vi "Serialize.vi"(0 "Input 6":variant, 4 "Input 5":variant, 6 "Input 4":variant, 8 "Input 3":variant, 9 "Input 2":variant, 10 "Input 1":variant, 11 "Base Actor in":refnum<class "Base Actor.lvclass">) -> (3 "Base Actor out":refnum<class "Base Actor.lvclass">)   [LabVIEW 2021, in "jettl.lvlib" / "Actor.lvlib" / "Base Actor.lvclass"]
uses:
  Base Actor.lvclass
  Base Actor.lvclass/Base Actor.ctl
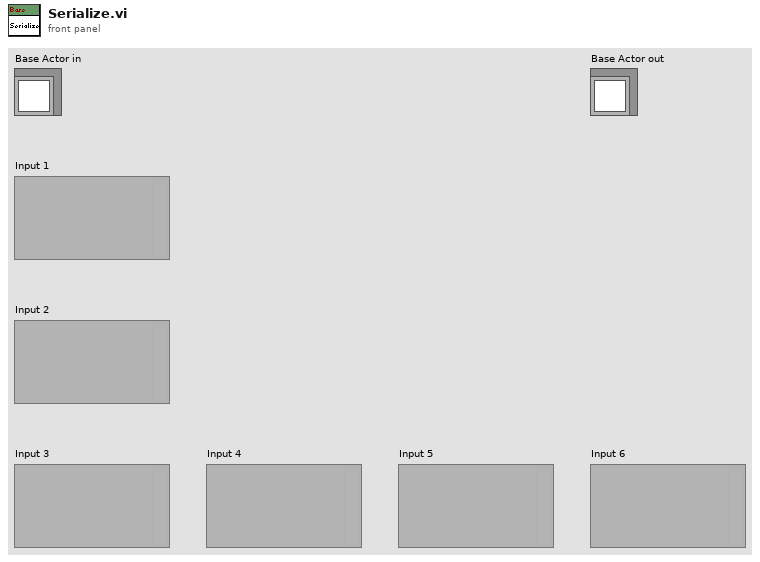
[diagram p1: front panel]
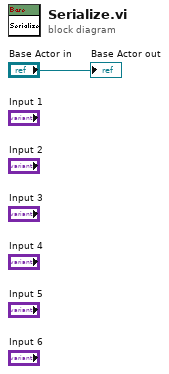
[diagram p0: block diagram]
diagram:
  "Base Actor out" <- "Base Actor in"
